vi "Button Digital Panel.vi"() -> ()   [LabVIEW 2020, in "VolatusGUI.lvlib" / "Telemetry Command Module.lvclass"]
uses:
  Telemetry Command Module.lvclass
  Telemetry Command Module.lvclass/Telemetry Command Module.ctl
panel:
  in  "Button":cluster{"Color":u32, "Button":bool}
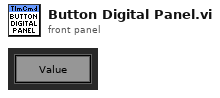
[diagram p1: front panel]
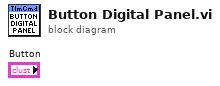
[diagram p0: block diagram]
diagram:
